vi "Queues vs Local Variables.vi"() -> ()   [LabVIEW 2010]
panel:
  in  "Loop Time (ms)":u16(ring)=50 caption="Loop Speed" items=["Same as Producer Loop"=50, "Maximum Speed"=0, "2x as Producer"=25, "1/2 as Producer"=100, "1/20 as Producer"=1000]
  out "Difference in Points":i32 caption="Duplicate Points"
  in  "Loop Time (ms)":u16(ring)=50 caption="Loop Speed" items=["Same as Producer Loop"=50, "Maximum Speed"=0, "2x as Producer"=25, "1/2 as Producer"=100, "1/20 as Producer"=1000]
  out "# of elements in queue":i32(slide) scale=0.0..1000.0
  out "# of points generated\nby Producer Loop":i32 caption="# of points generated by Producer Loop"
  in  "stop":bool
  out "Local Variables Consumer Loop":dbl(graph) caption="Sine"
  out "Queues Consumer Loop":dbl(graph)=-9.510565162951542 caption="Sine"
  out "Producer Loop":dbl(graph) caption="Sine"
  # "Producer Loop"
  # "Loop Time = 50 ms"
  # "Local Variables Consumer Loop"
  # "Queues Consumer Loop"
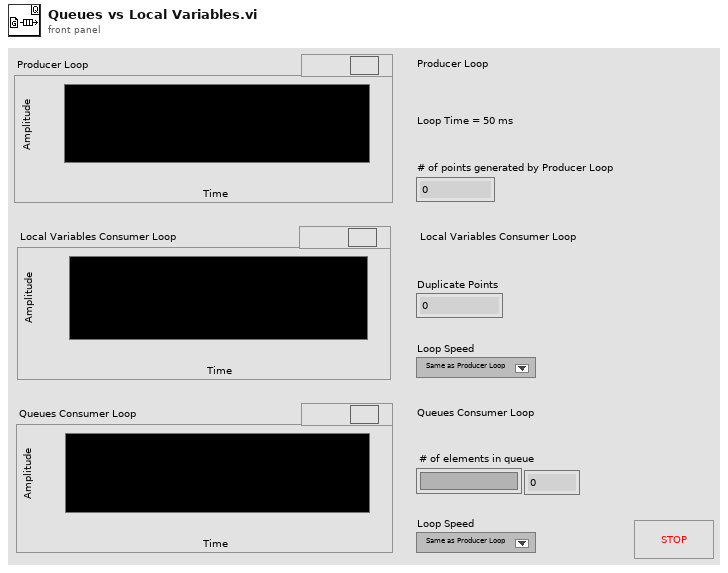
[diagram p1: front panel]
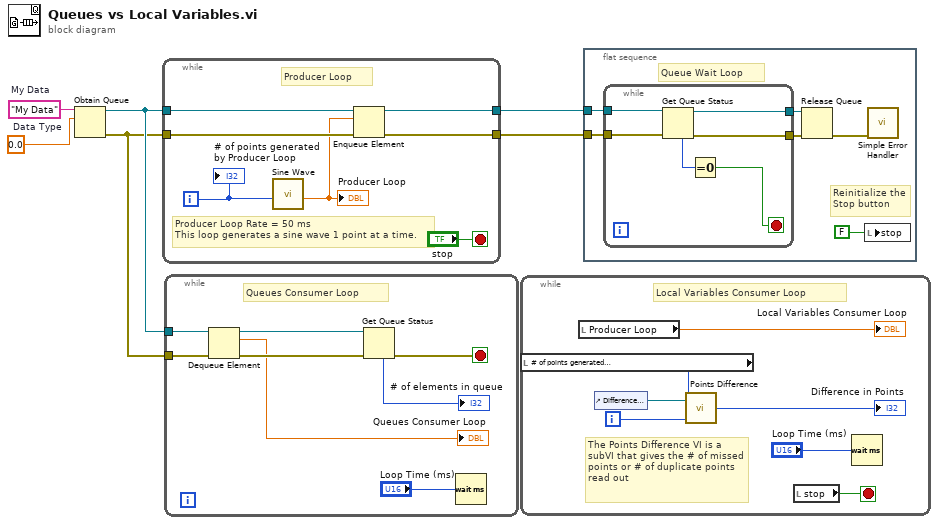
[diagram p0: block diagram]
diagram:
  w5 = "My Data"  # My Data
  w6 = 0.0  # Data Type
  n1 = Obtain Queue(name (unnamed)=w5, element data type=w6) -> (queue out=w4:refnum<queue>, error out=w1:errorcluster)  [unwired: 3 in, 1 out]
  n2 = while {
    tunnel: w4 -> [w11]
    tunnel: w1 -> [w10]
    tunnel: [w8] -> w3
    tunnel: [w7] -> w2
    i -> [w12]
    stop <- "stop" stop-if-true
    # "Producer Loop"
    # "Producer Loop Rate = 50 ms\nThis loop generates a sine wave 1 point at a time."
    n3 = call "Sine Wave.vi"("Numeric"=w12) -> ("Sine Wave"=w9:dbl)  [unwired: 6 out]
    "Producer Loop" <- w9
    n4 = Enqueue Element(queue=w11, element=w9, error in (no error)=w10) -> (queue out=w7:refnum<queue>, error out=w8:errorcluster)  [unwired: 2 out]
    "# of points generated\nby Producer Loop" <- w12
  }
  n5 = while {
    tunnel: w4 -> [w18]
    tunnel: w1 -> [w17]
    stop <- w15 stop-if-true
    # "Queues Consumer Loop"
    n6 = Dequeue Element(queue=w18, error in (no error)=w17) -> (queue out=w20:refnum<queue>, element=→"Queues Consumer Loop":dbl, error out=w19:errorcluster)  [unwired: 2 out]
    n7 = Get Queue Status(queue=w20, error in (no error)=w19) -> (error out=w15:errorcluster, # elements in queue=→"# of elements in queue":i32)  [unwired: 1 in, 6 out]
    n8 = Wait (ms)(milliseconds to wait="Loop Time (ms)") -> ()  [unwired: 1 out]
  }
  n9 = while {
    i -> [w26]
    stop <- w22 stop-if-true
    # "Local Variables Consumer Loop"
    # "The Points Difference VI is a subVI that gives the # of missed points or # of duplicate points read out"
    n10 = local read "# of points generated\nby Producer Loop"() -> (w27:i32)
    n11 = local read "Producer Loop"() -> (→"Local Variables Consumer Loop":dbl)
    n12 = control-ref of="Difference in Points"() -> (w23:refnum<vi>)
    n13 = call "Points Difference.vi"("# of Points (Consumer Loop)"=w26, "Points Missed Control Refnuma"=w23, "# of Points (Producer Loop)"=w27) -> ("Points Missed"=→"Difference in Points":i32)
    n14 = local read "stop"() -> (w22:bool)
    n15 = Wait (ms)(milliseconds to wait="Loop Time (ms)") -> ()  [unwired: 1 out]
  }
  n16 = flat-sequence {
    tunnel: w3 -> [w31]
    tunnel: w2 -> [w32]
    frame #0 {
      # "Queue Wait Loop"
      # "Reinitialize the\nStop button"
      n17 = while {
        tunnel: w32 -> [w40]
        tunnel: w31 -> [w39]
        tunnel: [w38] -> w30
        tunnel: [w37] -> w29
        stop <- w35 stop-if-true
        n18 = Get Queue Status(queue=w40, error in (no error)=w39) -> (queue out=w37:refnum<queue>, error out=w38:errorcluster, # elements in queue=w36:i32)  [unwired: 6 out]
        n19 = Equal To 0?(x=w36) -> (x = 0?=w35:bool)
      }
      n20 = Release Queue(queue=w29, error in (no error)=w30) -> (error out=w33:errorcluster)  [unwired: 3 out]
      n21 = local write "stop"(FALSE ("stop")) -> ()
      n22 = call <vilib>:"Simple Error Handler.vi"("error in (no error)"=w33) -> ()  [unwired: 2 in, 7 out]
    }
  }
